vi "Auto Shift.vi"(8 "Auto Shift Settings":T1={"Enabled"=FALSE, "Upshift Speed"=6.0, "Downshift Speed"=3.0, "Upshift Throttle"=0.6000000000000001, "Turn Power Diff"=0.7, "Motor Limit"=400.0, "Encoder Limit"=100.0}, 10 "Encoder Values":T2, 11 "Drive Controls":T3) -> (3 "Low gear output":bool)   [LabVIEW 2013]
uses:
  Encoder Values.ctl
  Auto Shift Settings.ctl
  <vilib>/addons/control/pid/pid.llb/PID Output Rate Limiter (DBL Array).vi
  <vilib>/addons/control/pid/NI_PID_pid.lvlib
panel:
  in  "Reset":bool
  in  "Zoom":dbl(slide) scale=0.0..10.0
  in  "Scroll":dbl(slide) scale=0.0..10.0
  out "Turn":bool
  out "Motor Power":dbl[][](graph)
  out "Encoders":dbl[][](graph)
  out "Low Speed":bool
  out "Accelerating":bool
  out "Low gear":bool
  in  "Graph":bool
  out "Waveform Chart":dbl[][](graph)
  out "High gear":bool
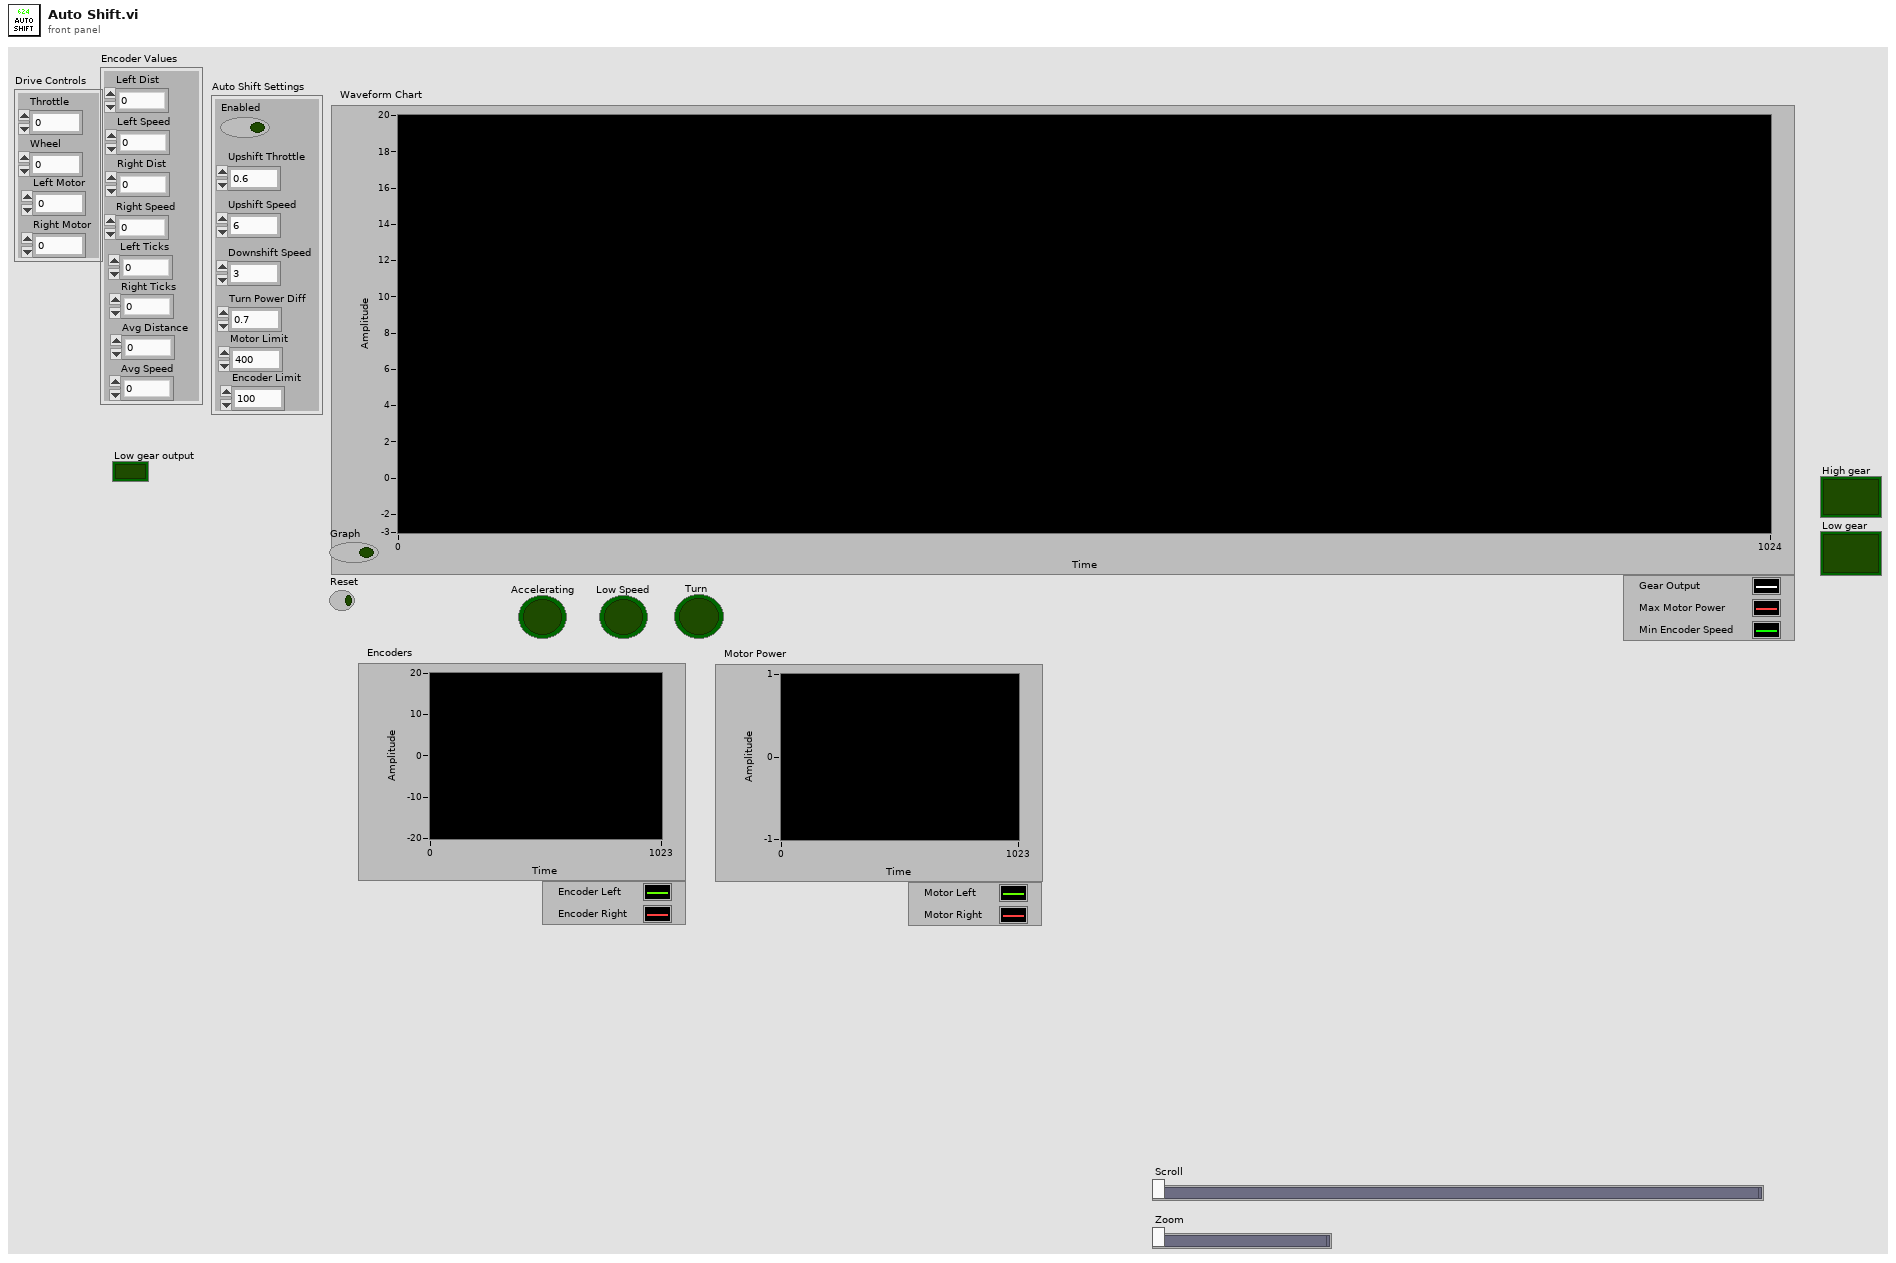
[diagram p1: front panel]
types:
  T1 = typedef "Auto Shift Settings.ctl" = cluster{"Enabled":bool, "Upshift Speed":dbl, "Downshift Speed":dbl, "Upshift Throttle":dbl, "Turn Power Diff":dbl, "Motor Limit":dbl, "Encoder Limit":dbl}
  T2 = typedef "Encoder Values.ctl" = cluster{"Left Dist":dbl, "Left Speed":dbl, "Right Dist":dbl, "Right Speed":dbl, "Left Ticks":dbl, "Right Ticks":dbl, "Avg Distance":dbl, "Avg Speed":dbl}
  T3 = cluster{"Throttle":dbl, "Wheel":dbl, "Right Motor":dbl, "Left Motor":dbl}
  T4 = typedef "Auto Shift Settings.ctl" = cluster{"Enabled":bool, "Upshift Speed":dbl, "Downshift Speed":dbl, "Throttle Mode":bool, "Upshift Throttle":dbl, "Downshift Throttle":dbl}
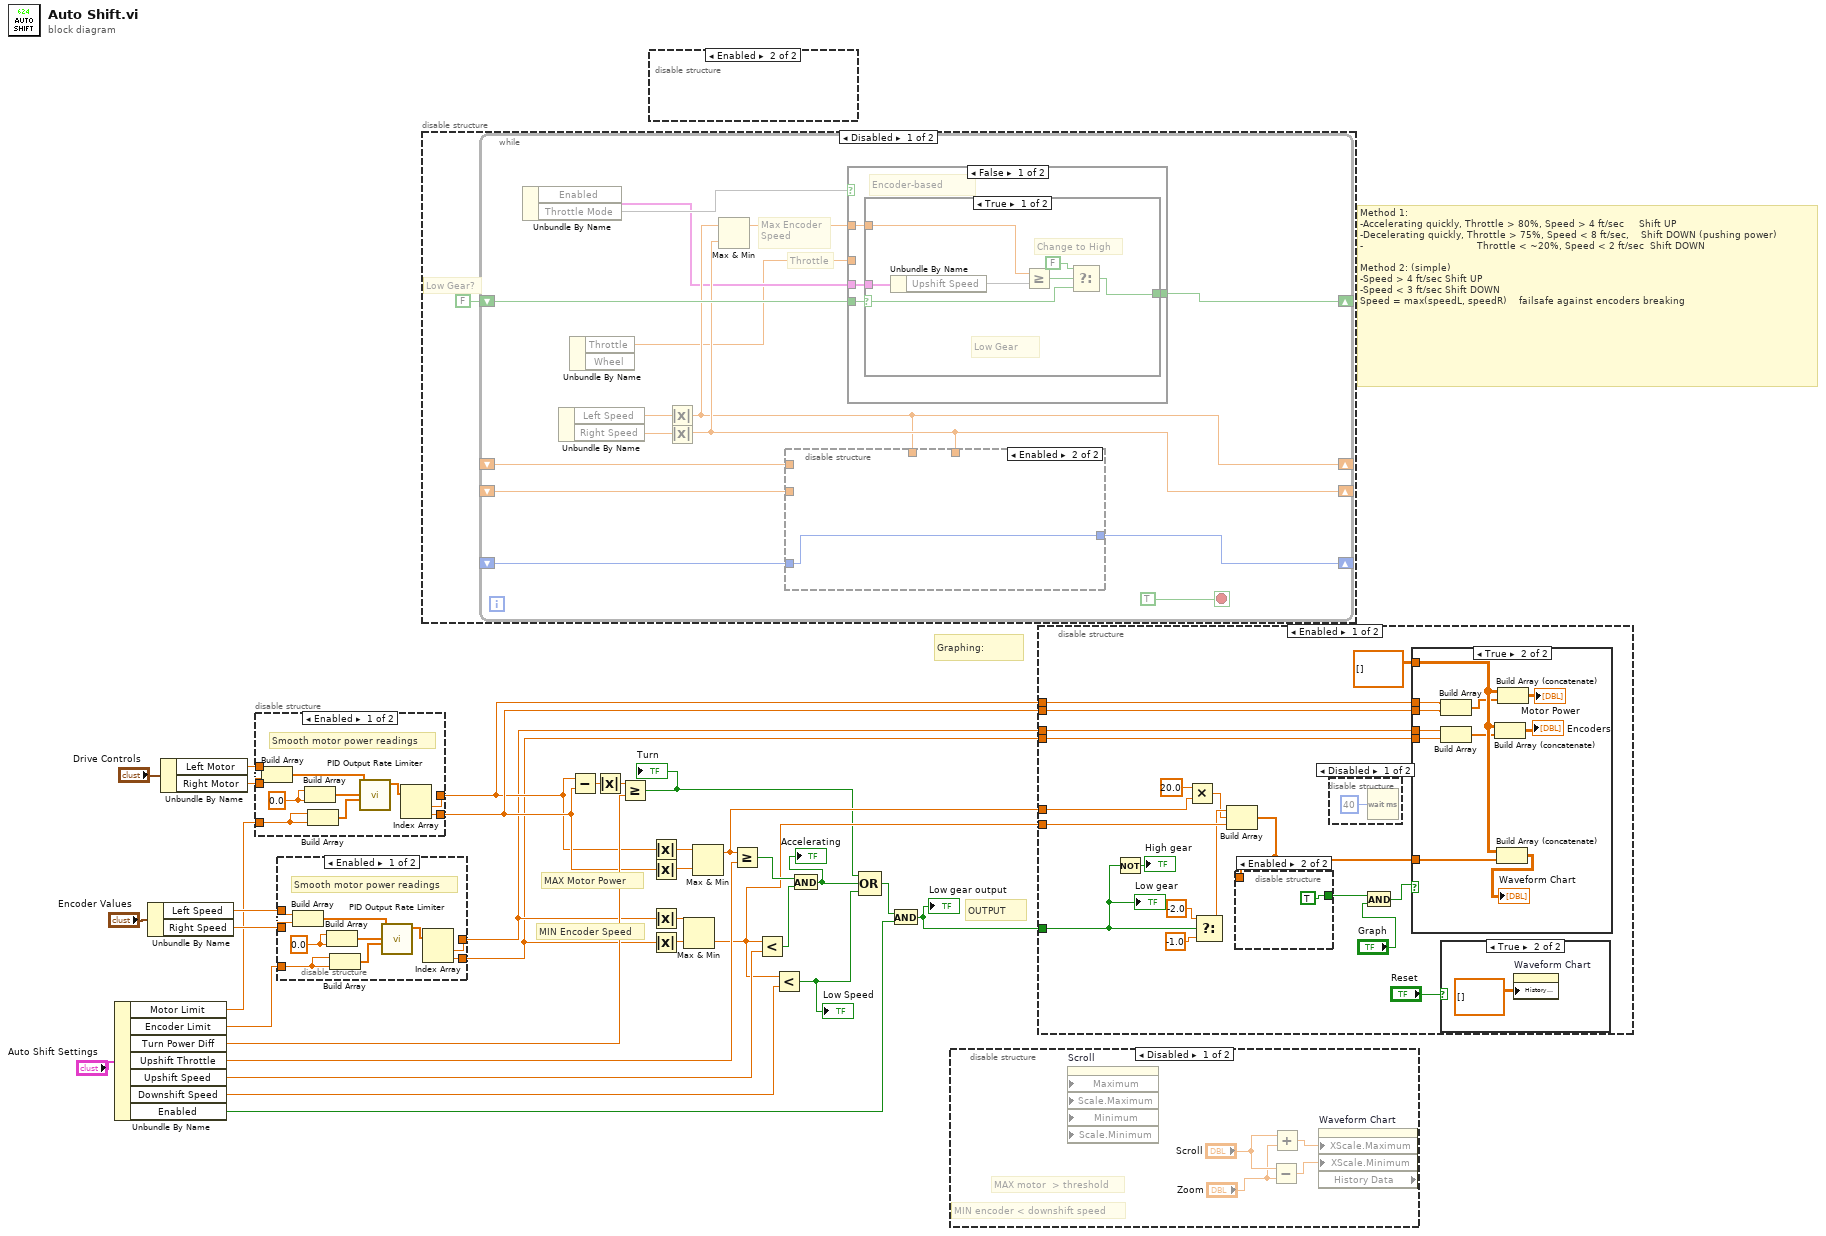
[diagram p0: block diagram]
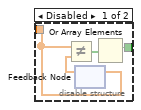
[diagram p7: hidden frame]
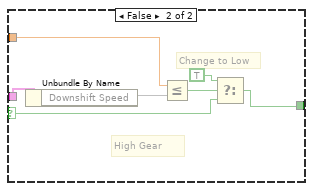
[diagram p10: hidden frame]
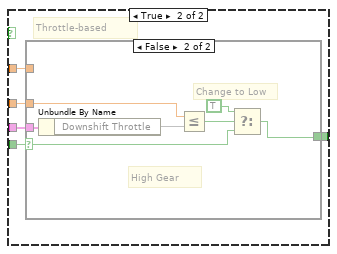
[diagram p11: hidden frame]
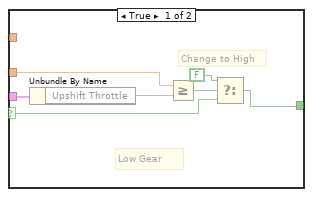
[diagram p12: hidden frame]
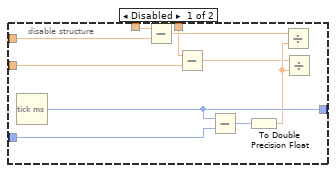
[diagram p13: hidden frame]
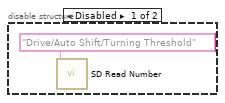
[diagram p15: hidden frame]
diagram:
  # "OUTPUT"
  # "Graphing:"
  # "MAX Motor Power"
  # "MIN Encoder Speed"
  # "Method 1:\n-Accelerating quickly, Throttle > 80%, Speed > 4 ft/sec     Shift UP\n-Decelerating quickly, Throttle > 75%, Speed < 8 ft/sec,    Shift DOWN (pushing power)\n-                                      Throttle < ~20%, Speed < 2 ft/sec  Shift DOWN\n\nMethod 2: (simple)\n-Speed > 4 ft/sec Shift UP\n-Speed < 3 ft/sec Shift DOWN\nSpeed = max(speedL, speedR)    failsafe against encoders breaking"
  n1 = Unbundle By Name("Auto Shift Settings") -> ("Motor Limit"=w2:dbl, "Encoder Limit"=w1:dbl, "Turn Power Diff"=w17:dbl, "Upshift Throttle"=w30:dbl, "Upshift Speed"=w27:dbl, "Downshift Speed"=w25:dbl, "Enabled"=w21:bool)
  n2 = Unbundle By Name("Encoder Values") -> ("Left Speed"=w4:dbl, "Right Speed"=w3:dbl)
  n3 = Unbundle By Name("Drive Controls") -> ("Left Motor"=w12:dbl, "Right Motor"=w10:dbl)
  n4 = disable-structure shown="Enabled" {
    disable-tunnel: w12 -> [w38 _]
    disable-tunnel: [w37 _] -> w11
    disable-tunnel: w10 -> [w36 _]
    disable-tunnel: [w35 _] -> w9
    disable-tunnel: w2 -> [w34 _]
    frame Enabled {
      w40 = 0.0 ("initial output")
      # "Smooth motor power readings"
      n5 = Build Array(w38, w36) -> (w39:dbl[])
      n6 = Build Array(w40, w40) -> (w41:dbl[])
      n7 = Build Array(w34, w34) -> (w42:dbl[])
      n8 = call-poly <vilib>:"PID Output Rate Limiter.vi"("output rate (EGU/min)"=w42, "initial output"=w41, "input (controller output)"=w39) -> ("output"=w43:dbl[])  [unwired: 5 in, 1 out]
      n9 = Index Array(array=w43) -> (element #1=w35:dbl, element #2=w37:dbl)  [unwired: 2 in]
    }
    frame Disabled {
    }
  }
  n10 = disable-structure shown="Enabled" {
    disable-tunnel: w4 -> [w48 _]
    disable-tunnel: [w47 _] -> w5
    disable-tunnel: w3 -> [w46 _]
    disable-tunnel: [w45 _] -> w6
    disable-tunnel: w1 -> [w44 _]
    frame Enabled {
      w50 = 0.0 ("initial output")
      # "Smooth motor power readings"
      n11 = Build Array(w48, w46) -> (w49:dbl[])
      n12 = Build Array(w50, w50) -> (w51:dbl[])
      n13 = Build Array(w44, w44) -> (w52:dbl[])
      n14 = call-poly <vilib>:"PID Output Rate Limiter.vi"("output rate (EGU/min)"=w52, "initial output"=w51, "input (controller output)"=w49) -> ("output"=w53:dbl[])  [unwired: 5 in, 1 out]
      n15 = Index Array(array=w53) -> (element #1=w45:dbl, element #2=w47:dbl)  [unwired: 2 in]
    }
    frame Disabled {
    }
  }
  n16 = disable-structure shown="Disabled" {
    frame Disabled {
      # "Low Gear?"
      n17 = while {
        shift-right: [w63] -> _
        shift-left: _ -> [w68]
        shift-right: [w62] -> _
        shift-left: _ -> [w69]
        shift-right: [w67] -> _
        shift-left: _ -> [w66]
        shift-right: [w58] -> _
        shift-left: FALSE ("Shifter Output") -> [w65]
        stop <- TRUE stop-if-true
        # "Throttle"
        # "Max Encoder\nSpeed"
        n18 = Unbundle By Name() -> (w56:T4, "Enabled"=w59, "Throttle Mode"=w57)
        n19 = Unbundle By Name() -> ("Left Speed"=w61:dbl, "Right Speed"=w60:dbl)  [unwired: 1 in]
        n20 = Unbundle By Name() -> ("Throttle"=w55:dbl)  [unwired: 1 in, 1 out]
        n21 = Absolute Value(x=w61) -> (abs(x)=w62:dbl)
        n22 = Absolute Value(x=w60) -> (abs(x)=w63:dbl)
        n23 = Max & Min(x=w62, y=w63) -> (max(x,y)=w64:dbl)  [unwired: 1 out]
        n24 = disable-structure shown="Enabled" {
          disable-tunnel: w69 -> [w117 _]
          disable-tunnel: w68 -> [w116 _]
          disable-tunnel: [w115 w118] -> w67
          disable-tunnel: w66 -> [w114 w118]
          disable-tunnel: w63 -> [w109 _]
          disable-tunnel: w62 -> [w108 _]
          frame Disabled {
            n25 = Tick Count (ms)() -> (millisecond timer value=w115:u32)
            n26 = Subtract(x=w108, y=w117) -> (x-y=w110:dbl)
            n27 = Subtract(x=w109, y=w116) -> (x-y=w111:dbl)
            n28 = Subtract(x=w115, y=w114) -> (x-y=w113:u32)
            n29 = To Double Precision Float(number=w113) -> (double precision float=w112:dbl)
            n30 = Divide(x=w110, y=w112) -> ()  [unwired: 1 out]
            n31 = Divide(x=w111, y=w112) -> ()  [unwired: 1 out]
          }
          frame Enabled {
          }
        }
        n32 = case shown="False" w57 {
          tunnel: w65 -> [w74 w93]
          tunnel: w64 -> [w73 w92]
          tunnel: [w72 w91] -> w58
          tunnel: w56 -> [w71 w90]
          tunnel: w55 -> [_ w89]
          frame False {
            # "Encoder-based"
            n33 = case shown="True" w74 {
              selector: w74 -> [w78 w85]
              tunnel: w73 -> [w81 w88]
              tunnel: [w79 w86] -> w72
              tunnel: w71 -> [w76 w83]
              frame True {
                # "Low Gear"
                # "Change to High"
                n34 = Unbundle By Name(w76) -> ("Upshift Speed"=w75)
                n35 = Greater Or Equal?(x=w81, y=w75) -> (x >= y?=w77:bool)
                n36 = Select(t=FALSE ("Shifter Output"), s=w77, f=w78) -> (s? t:f=w79:bool)
              }
              frame False {
                # "Change to Low"
                # "High Gear"
                n37 = Unbundle By Name(w83) -> ("Downshift Speed"=w82)
                n38 = Less Or Equal?(x=w88, y=w82) -> (x <= y?=w84:bool)
                n39 = Select(t=TRUE ("Shifter Output"), s=w84, f=w85) -> (s? t:f=w86:bool)
              }
            }
          }
          frame True {
            # "Throttle-based"
            n40 = case shown="False" w93 {
              selector: w93 -> [w98 w105]
              tunnel: w92 -> [_ _]
              tunnel: [w99 w106] -> w91
              tunnel: w90 -> [w96 w103]
              tunnel: w89 -> [w94 w101]
              frame True {
                # "Low Gear"
                # "Change to High"
                n41 = Unbundle By Name(w96) -> ("Upshift Throttle"=w95)
                n42 = Greater Or Equal?(x=w94, y=w95) -> (x >= y?=w97:bool)
                n43 = Select(t=FALSE ("Shifter Output"), s=w97, f=w98) -> (s? t:f=w99:bool)
              }
              frame False {
                # "Change to Low"
                # "High Gear"
                n44 = Unbundle By Name(w103) -> ("Downshift Throttle"=w102)
                n45 = Less Or Equal?(x=w101, y=w102) -> (x <= y?=w104:bool)
                n46 = Select(t=TRUE ("Shifter Output"), s=w104, f=w105) -> (s? t:f=w106:bool)
              }
            }
          }
        }
      }
    }
    frame Enabled {
    }
  }
  n47 = Subtract(x=w9, y=w11) -> (x-y=w8:dbl)
  n48 = Absolute Value(x=w8) -> (abs(x)=w7:dbl)
  n49 = Greater Or Equal?(x=w7, y=w17) -> (x >= y?=w13:bool)
  "Turn" <- w13
  n50 = disable-structure shown="Enabled" {
    frame Disabled {
      n51 = call <vilib>:"SD Read Number.vi"("Name"="Drive/Auto Shift/Turning Threshold") -> ("Numeric"=w119:dbl)  [unwired: 8 in, 2 out]
    }
    frame Enabled {
    }
  }
  n52 = Absolute Value(x=w9) -> (abs(x)=w23:dbl)
  n53 = Absolute Value(x=w11) -> (abs(x)=w22:dbl)
  n54 = Absolute Value(x=w6) -> (abs(x)=w24:dbl)
  n55 = Absolute Value(x=w5) -> (abs(x)=w28:dbl)
  n56 = Max & Min(x=w24, y=w28) -> (min(x,y)=w20:dbl)  [unwired: 1 out]
  n57 = Max & Min(x=w23, y=w22) -> (max(x,y)=w18:dbl)  [unwired: 1 out]
  n58 = Greater Or Equal?(x=w18, y=w30) -> (x >= y?=w29:bool)
  n59 = Less?(x=w20, y=w27) -> (x < y?=w26:bool)
  n60 = Less?(x=w20, y=w25) -> (x < y?=w16:bool)
  "Low Speed" <- w16
  n61 = And(x=w29, y=w26) -> (x .and. y?=w15:bool)
  "Accelerating" <- w15
  n62 = Compound Arithmetic op=OR(w13, w15, w16) -> (w14:bool)
  n63 = And(x=w14, y=w21) -> (x .and. y?=w19:bool)
  "Low gear output" <- w19
  n64 = disable-structure shown="Disabled" {
    frame Disabled {
      # "MAX motor  > threshold"
      # "MIN encoder < downshift speed"
      n65 = property on="Scroll" class="Slide (strict)" props=["Maximum", "Scale", "Maximum", "Minimum", "Scale", "Minimum"]() -> ()  [unwired: 6 in, 2 out]
      n66 = Subtract(x="Scroll", y="Zoom") -> (x-y=w123:dbl)
      n67 = Add(x="Scroll", y="Zoom") -> (x+y=w124:dbl)
      n68 = property on="Waveform Chart" class="WFChart (strict)" props=["XScale", "Maximum", "XScale", "Minimum", "History Data"]("XScale.Maximum"=w124, "XScale.Minimum"=w123) -> ()  [unwired: 2 in, 3 out]
    }
    frame Enabled {
    }
  }
  n69 = disable-structure shown="Enabled" {
    disable-tunnel: w20 -> [w142 _]
    disable-tunnel: w18 -> [w132 _]
    disable-tunnel: w19 -> [w133 _]
    disable-tunnel: w9 -> [w129 _]
    disable-tunnel: w11 -> [w130 _]
    disable-tunnel: w6 -> [w128 _]
    disable-tunnel: w5 -> [w127 _]
    frame Enabled {
      n70 = Not(x=w133) -> (.not. x?=→"High gear":bool)
      n71 = Multiply(x=20.0 ("y"), y=w132) -> (x*y=w137:dbl)
      n72 = Select(t=-2.0, s=w133, f=-1.0) -> (s? t:f=w139:dbl)
      n73 = Build Array(w139, w137, w142) -> (w136:dbl[])
      n74 = disable-structure shown="Enabled" {
        disable-tunnel: w136 -> [w149 _]
        disable-tunnel: [w146 TRUE] -> w135
        frame Disabled {
          n75 = feedback #1() -> (w147:dbl[])  [unwired: 1 in]
          n76 = Not Equal?(x=w149, y=w147) -> (x != y?=w148:bool[])
          n77 = feedback-in #1(w149) -> ()
          n78 = Or Array Elements(Boolean array=w148) -> (logical OR=w146:bool)
        }
        frame Enabled {
        }
      }
      n79 = disable-structure shown="Disabled" {
        frame Disabled {
          n80 = Wait (ms)(milliseconds to wait=u32 40) -> ()  [unwired: 1 out]
        }
        frame Enabled {
        }
      }
      n81 = And(x=w135, y="Graph") -> (x .and. y?=w134:bool)
      n82 = case shown="True" w134 {
        tunnel: w136 -> [_ w161]
        tunnel: dbl[][] [] ("appended array") -> [_ w157]
        tunnel: w130 -> [_ w155]
        tunnel: w129 -> [_ w154]
        tunnel: w128 -> [_ w153]
        tunnel: w127 -> [_ w152]
        frame False {
        }
        frame True {
          n83 = Build Array(w154, w155) -> (w156:dbl[])
          n84 = Build Array(w153, w152) -> (w151:dbl[])
          n85 = Build Array (concatenate)(w157, w151) -> (→"Encoders":dbl[][])
          n86 = Build Array (concatenate)(w157, w161) -> (→"Waveform Chart":dbl[][])
          n87 = Build Array (concatenate)(w157, w156) -> (→"Motor Power":dbl[][])
        }
      }
      n88 = case shown="True" "Reset" {
        frame False {
        }
        frame True {
          n89 = property on="Waveform Chart" class="WFChart (strict)"("History Data"=dbl[][] []) -> ()  [unwired: 2 in, 2 out]
        }
      }
      "Low gear" <- w133
    }
    frame Disabled {
    }
  }
